vi "Add File Exists Checker.vi"(11 "Response Handler Map In":T1) -> (3 "Response Handler Map":T1)   [LabVIEW 2020, in "HTTP Server.lvlib" / "Server.lvclass"]
uses:
  Server.lvclass
  FileExistChecker/FileExistChecker.lvclass
  Response Handler/Response Handler.lvclass
  Priority.ctl
  HTTP Server.lvlib
  Response Handler Map.ctl
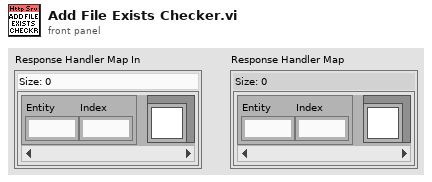
[diagram p1: front panel]
types:
  T1 = typedef "HTTP Server.lvlib/Response Handler Map.ctl" = map{T2, refnum<class "Response Handler.lvclass">}
  T2 = typedef "HTTP Server.lvlib/Priority.ctl" = cluster{"Entity":u16, "Index":u16}
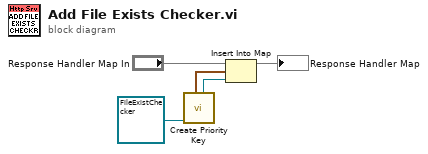
[diagram p0: block diagram]
diagram:
  n1 = call "Create Priority Key.vi"("Handler In"=refnum<class "FileExistChecker.lvclass"> refnum ("HTTP Server.lvlib:FileExistChecker.lvclass")) -> ("Handler"=w4:refnum<class "FileExistChecker.lvclass">, "Priority Key"=w5:T2)  [unwired: 8 in, 1 out]
  n2 = Insert Into Map(map in="Response Handler Map In", key=w5, value=w4) -> (map out=→"Response Handler Map":T1)  [unwired: 2 out]
